vi "AgB29xx_LabVIEW_FixedDC.vi"() -> ()   [LabVIEW 2009]
panel:
  out "Items":string
  out "Simulate":bool
  out "SerialNumber":string
  out "Identifier":string
  out "Revision":string
  out "Vendor":string
  out "Description":string
  out "InstrumentModel":string
  out "InstrumentFirmwareRevision":string
  in  "OptionString":string="QueryInstrStatus=true, Simulate=true, DriverSetup= Model=, Trace=false"
  in  "Reset":bool=TRUE
  in  "IdQuery":bool=TRUE
  in  "ResourceName":string="GPIB0::23::INSTR"
  out "iNumberOfChannels":i32=2
  out "data":dbl[](array[numeric])
  in  "AgB29xxLib.IAgB29xx2":refnum<k7>
  # "FixedDC"
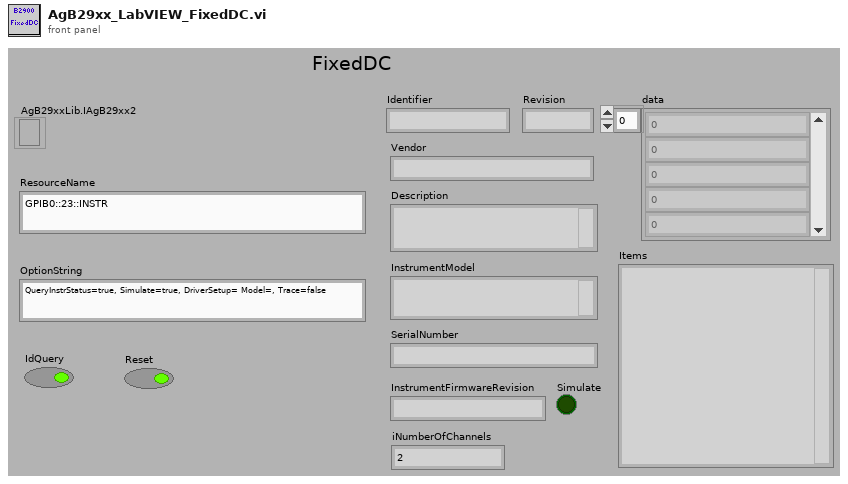
[diagram p1: front panel]
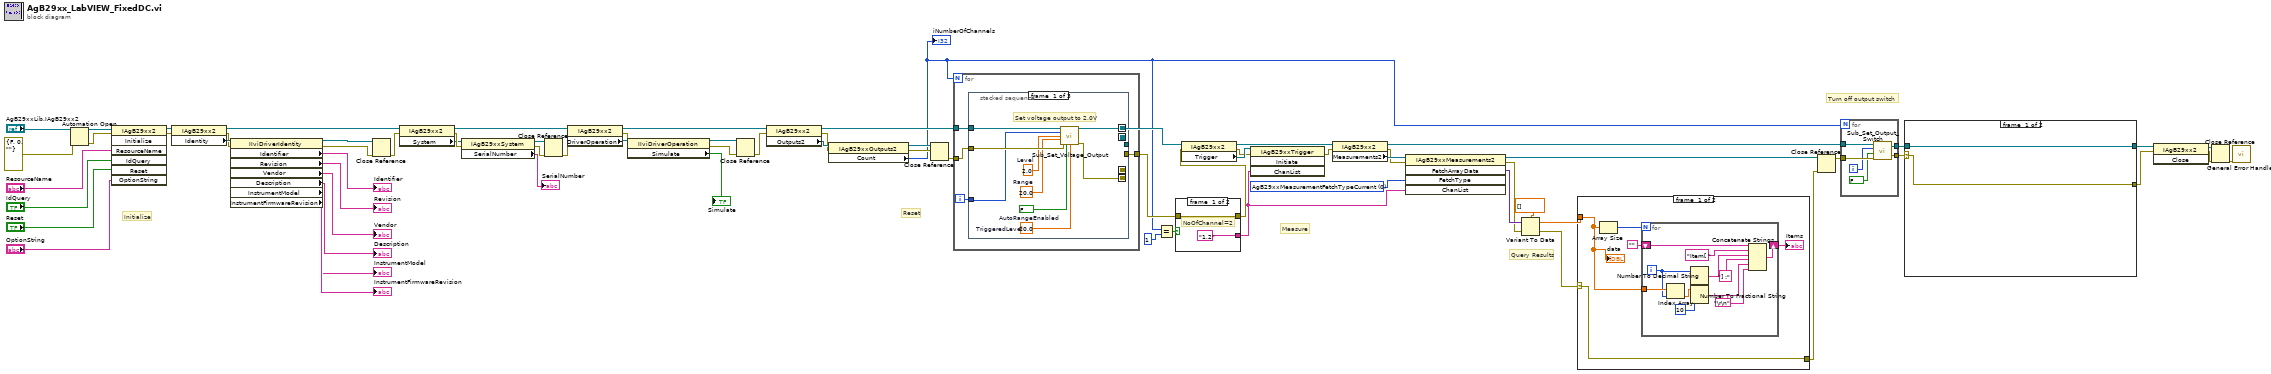
[diagram p0: block diagram]
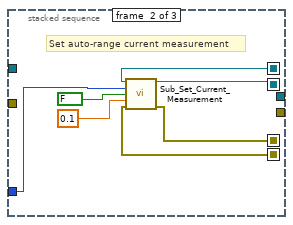
[diagram p2: hidden frame]
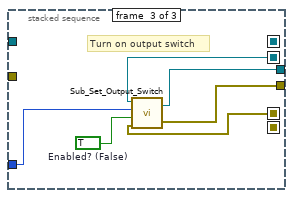
[diagram p3: hidden frame]
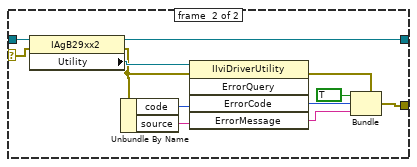
[diagram p4: hidden frame]
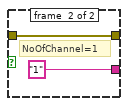
[diagram p6: hidden frame]
diagram:
  w61 = 0 items=["AgB29xxMeasurementFetchTypeCurrent", "AgB29xxMeasurementFetchTypeResistance", "AgB29xxMeasurementFetchTypeSource", "AgB29xxMeasurementFetchTypeStatus", "AgB29xxMeasurementFetchTypeTime", "AgB29xxMeasurementFetchTypeVoltage", "AgB29xxMeasurementFetchTypeAll"] ("FetchType")
  # "Turn off output switch"
  # "Query Results"
  # "Measure"
  # "Initialize"
  # "Reset"
  n1 = Automation Open(error in (no error)=errorcluster {"status"=FALSE, "code"=0, "source"=""}, Automation Refnum="AgB29xxLib.IAgB29xx2") -> (Automation Refnum=w47:refnum<k7>, error out=w69:errorcluster)  [unwired: 2 in]
  n2 = invoke class="IAgB29xx2" method="Initialize"(reference=w47, error in=w69, "ResourceName"="ResourceName", "IdQuery"="IdQuery", "Reset"="Reset", "OptionString"="OptionString") -> (reference out=w45:refnum<k7>, error out=w40:errorcluster)  [unwired: 1 in, 5 out]
  n3 = property class="IAgB29xx2"(reference=w45, error in=w40) -> (reference out=w41:refnum<k7>, error out=w43:errorcluster, "Identity"=w44:refnum<k7>)
  n4 = property class="IIviDriverIdentity"(reference=w44, error in=w43) -> (reference out=w39:refnum<k7>, error out=w38:errorcluster, "Identifier"=→"Identifier":string, "Revision"=→"Revision":string, "Vendor"=→"Vendor":string, "Description"=→"Description":string, "InstrumentModel"=→"InstrumentModel":string, "InstrumentFirmwareRevision"=→"InstrumentFirmwareRevision":string)
  n5 = Close Reference(reference=w39, error in (no error)=w38) -> (error out=w37:errorcluster)
  n6 = property class="IAgB29xx2"(reference=w41, error in=w37) -> (reference out=w34:refnum<k7>, error out=w42:errorcluster, "System"=w1:refnum<k7>)
  n7 = property class="IAgB29xxSystem"(reference=w1, error in=w42) -> (reference out=w32:refnum<k7>, error out=w33:errorcluster, "SerialNumber"=→"SerialNumber":string)
  n8 = Close Reference(reference=w32, error in (no error)=w33) -> (error out=w31:errorcluster)
  n9 = property class="IAgB29xx2"(reference=w34, error in=w31) -> (reference out=w30:refnum<k7>, error out=w35:errorcluster, "DriverOperation"=w36:refnum<k7>)
  n10 = property class="IIviDriverOperation"(reference=w36, error in=w35) -> (reference out=w29:refnum<k7>, error out=w28:errorcluster, "Simulate"=→"Simulate":bool)
  n11 = Close Reference(reference=w29, error in (no error)=w28) -> (error out=w27:errorcluster)
  n12 = property class="IAgB29xx2"(reference=w30, error in=w27) -> (reference out=w48:refnum<k7>, error out=w16:errorcluster, "Outputs2"=w18:refnum<k7>)
  n13 = property class="IAgB29xxOutputs2"(reference=w18, error in=w16) -> (reference out=w17:refnum<k7>, error out=w15:errorcluster, "Count"=w2:i32)
  "iNumberOfChannels" <- w2
  n14 = Close Reference(reference=w17, error in (no error)=w15) -> (error out=w50:errorcluster)
  n15 = for {
    N: w2 -> [_]
    tunnel: w50 -> [w75]
    tunnel: w48 -> [w74]
    tunnel: [w73] -> w12
    i -> [w72]
    n16 = stacked-sequence {
      seq-local: [w81 _ _] -> [_ w91 _]
      seq-local: [w82 _ _] -> [_ w86 _]
      seq-local: [_ w85 _] -> [_ _ w97]
      seq-local: [_ w90 _] -> [_ _ w96]
      tunnel: w74 -> [w84 _ _]
      tunnel: w75 -> [w83 _ _]
      tunnel: w72 -> [w78 w87 w93]
      tunnel: [_ _ w95] -> w73
      tunnel: [_ _ w94] -> _
      frame #0 {
        w76 = 20.0  # TriggeredLevel
        w77 = FALSE  # AutoRangeEnabled
        w79 = 2.0  # Level
        w80 = 20.0  # Range
        # "Set voltage output to 2.0V"
        n17 = call "Sub_Set_Voltage_Output.vi"("AgB29xxLib.IAgB29xx2"=w84, "i"=w78, "Level"=w79, "Range"=w80, "error in"=w83, "AutoRangeEnabled"=w77, "TriggeredLevel"=w76) -> ("AgB29xxLib.IAgB29xx2 2"=w81:refnum<k7>, "error out"=w82:errorcluster)  [unwired: 7 in]
      }
      frame #1 {
        # "Set auto-range current measurement"
        n18 = call "Sub_Set_Current_Measurement.vi"("AgB29xxLib.IAgB29xx2"=w91, "i"=w87, "AutoRangeEnabled"=FALSE, "NPLC"=0.1, "error in"=w86) -> ("AgB29xxLib.IAgB29xx2 2"=w90:refnum<k7>, "error out"=w85:errorcluster)  [unwired: 9 in]
      }
      frame #2 {
        w92 = TRUE  # Enabled? (False)
        # "Turn on output switch"
        n19 = call "Sub_Set_Output_Switch.vi"("error in"=w97, "Enabled? (False)"=w92, "i"=w93, "AgB29xxLib.IAgB29xx2"=w96) -> ("error out"=w95:errorcluster, "AgB29xxLib.IAgB29xx2 2"=w94:refnum<k7>)
      }
    }
  }
  n20 = Equal?(x=w2, y=1 ("iStart")) -> (x = y?=w14:bool)
  n21 = case shown="False" w14 {
    tunnel: ["1,2" "1"] -> w10
    tunnel: w12 -> [w98 w100]
    tunnel: [w98 w100] -> w11
    frame #0 {
      # "NoOfChannel=2"
    }
    frame #1 {
      # "NoOfChannel=1"
    }
  }
  n22 = property class="IAgB29xx2"(reference=w48, error in=w11) -> (reference out=w63:refnum<k7>, error out=w58:errorcluster, "Trigger"=w65:refnum<k7>)
  n23 = invoke class="IAgB29xxTrigger" method="Initiate"(reference=w65, error in=w58, "ChanList"=w10) -> (error out=w62:errorcluster)  [unwired: 1 in, 3 out]
  n24 = property class="IAgB29xx2"(reference=w63, error in=w62) -> (reference out=w53:refnum<k7>, error out=w57:errorcluster, "Measurements2"=w64:refnum<k7>)
  n25 = invoke class="IAgB29xxMeasurements2" method="FetchArrayData"(reference=w64, error in=w57, "FetchType"=w61, "ChanList"=w10) -> (reference out=w55:refnum<k7>, error out=w49:errorcluster, "FetchArrayData"=w59:variant)  [unwired: 1 in, 2 out]
  n26 = Variant To Data(error in=w49, Variant=w59, type=dbl[] []) -> (error out=w8:errorcluster, data=w9:dbl[])
  n27 = case shown="No Error" w8 {
    selector: w8 -> [w104 w118]
    tunnel: w9 -> [w103 _]
    tunnel: [w104 w118] -> w7
    frame #0 {
      n28 = Array Size(array=w103) -> (size(s)=w102:i32)
      n29 = for {
        N: w102 -> [_]
        tunnel: w103 -> [w113]
        shift-right: [w110] -> w106
        shift-left: "" -> [w109]
        i -> [w108]
        n30 = Index Array(array=w113, index=w108) -> (element=w112:dbl)
        n31 = Number To Decimal String(number=w108) -> (decimal integer string=w116:string)  [unwired: 1 in]
        n32 = Number To Fractional String(number=w112, precision (6)=i16 10) -> (F-format string=w114:string)  [unwired: 2 in]
        n33 = Concatenate Strings(w109, "Item[ " ("string"), w116, "] :" ("string"), w114, "\r\n") -> (w110:string)
      }
      "Items" <- w106
      "data" <- w103
    }
    frame #1 {
    }
  }
  n34 = Close Reference(reference=w55, error in (no error)=w7) -> (error out=w52:errorcluster)
  n35 = for {
    N: w2 -> [_]
    tunnel: w53 -> [w124]
    tunnel: w52 -> [w123]
    tunnel: [w121] -> w6
    tunnel: [w120] -> w5
    i -> [w119]
    n36 = call "Sub_Set_Output_Switch.vi"("error in"=w123, "Enabled? (False)"=FALSE ("AutoRangeEnabled"), "i"=w119, "AgB29xxLib.IAgB29xx2"=w124) -> ("error out"=w121:errorcluster, "AgB29xxLib.IAgB29xx2 2"=w120:refnum<k7>)
  }
  n37 = case shown="Error" w6 {
    selector: w6 -> [w125 w137]
    tunnel: [w125 w127] -> w3
    tunnel: w5 -> [w126 w138]
    tunnel: [w126 w135] -> w4
    frame #0 {
    }
    frame #1 {
      n38 = property class="IAgB29xx2"(reference=w138, error in=w137) -> (reference out=w135:refnum<k7>, error out=w132:errorcluster, "Utility"=w136:refnum<k7>)
      n39 = Unbundle By Name(w132) -> ("code"=w134:i32, "source"=w133:string)
      n40 = invoke class="IIviDriverUtility" method="ErrorQuery"(reference=w136, error in=w132, "ErrorCode"=w134, "ErrorMessage"=w133) -> (error out=w128:errorcluster, "ErrorCode"=w131:i32, "ErrorMessage"=w130:string)  [unwired: 1 in, 2 out]
      n41 = Bundle(cluster=w128, "status"=TRUE, "code"=w131, "source"=w130) -> (w127:errorcluster)
    }
  }
  n42 = invoke class="IAgB29xx2" method="Close"(reference=w4, error in=w3) -> (reference out=w70:refnum<k7>, error out=w68:errorcluster)  [unwired: 1 in, 1 out]
  n43 = Close Reference(reference=w70, error in (no error)=w68) -> (error out=w51:errorcluster)
  n44 = call <vilib>:"General Error Handler.vi"("error in (no error)"=w51) -> ()  [unwired: 10 in, 5 out]
